vi "Init Device.vi"(7 "Layout Ref":refnum<vi>, 8 "error in (no error)":errorcluster, 10 "Chan# Array":i32[](array[numeric])=[4, 16] caption="#AOs [0,8]   #DOs [0,32]", 11 "NI Card in":refnum<class "NI Card.lvclass">) -> (0 "error out":errorcluster={"status"=TRUE, "code"=1055, "source"="Property Node in NI Card.lvclass:Init Device.vi"}, 3 "NI Card out":refnum<class "NI Card.lvclass">)   [LabVIEW 2013, in "NI Card.lvclass"]
doc: "Initialize the correct columns and their default appearance.\nUse the front panel to change default appearance of the device in the Add/Manage devices.\n\nThe (optional) Chan# Array, used for Old version loading, is [# AOs, # DOs]."
uses:
  NI Card.lvclass
  TypeDefs/DigitalColumnAppearCluster.ctl
  TypeDefs/ColumnAppearCluster.ctl
  ColumnVIs/Column/Column.lvclass
  ColumnVIs/DigitalCol/DigitalCol.lvclass
  NI Card.lvclass/NI Card.ctl
panel:
  in  "AI Default Name":string
  in  "Analog Column Defaults":T1={"Column Name"="", "Width"=30, "Bkgd"=[16448250], "Text"=[0]}
  in  "Num AIs":i32
  in  "Digital Column Defaults":T2={"Column Name"="", "Width"=15, "Bkgd"=[1985280, 6618880, 14090026], "Text"=[16448250, 0, 0]}
  # "Num AOs, DOs are coerced on Block diagram to be in shown range.\nMUST include at least 1 to configure each column type."
  # "The choices you make here dictate what will appear when you Add an 'NI card' device.\nPick default widths, colors, (column names) and numbers of channels.\nThen go to the menu Edit >> Make Current Values Default and re-save the VI."
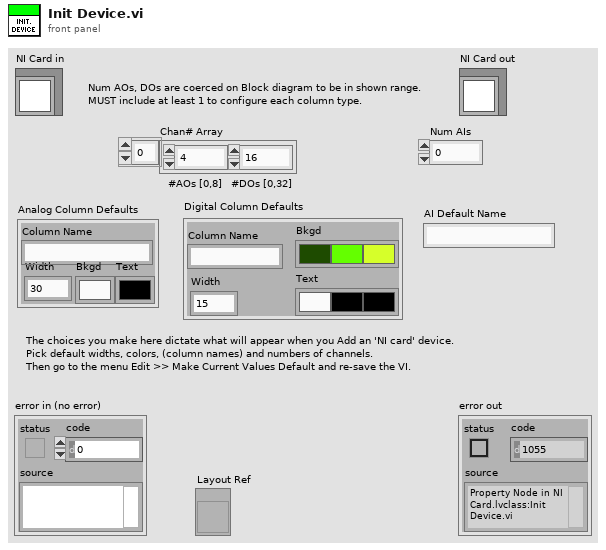
[diagram p1: front panel]
types:
  T1 = typedef "ColumnAppearCluster.ctl" = cluster{"Column Name":string, "Width":u32, "Bkgd":u32[], "Text":u32[]}
  T2 = typedef "DigitalColumnAppearCluster.ctl" = cluster{"Column Name":string, "Width":u32, "Bkgd":u32[], "Text":u32[]}
  T3 = cluster{"DAQmx Global Channel":refnum<k21>, "AI Default Name":string}
  T4 = cluster{"DAQmx Global Channel":refnum<k21>, "Column Name":string}
  T5 = cluster{"DAQmx Global Channel":refnum<k21>, "Column Name":string}[]
  T6 = cluster{"DAQmx Global Channel":refnum<k21>, "AI Default Name":string}[]
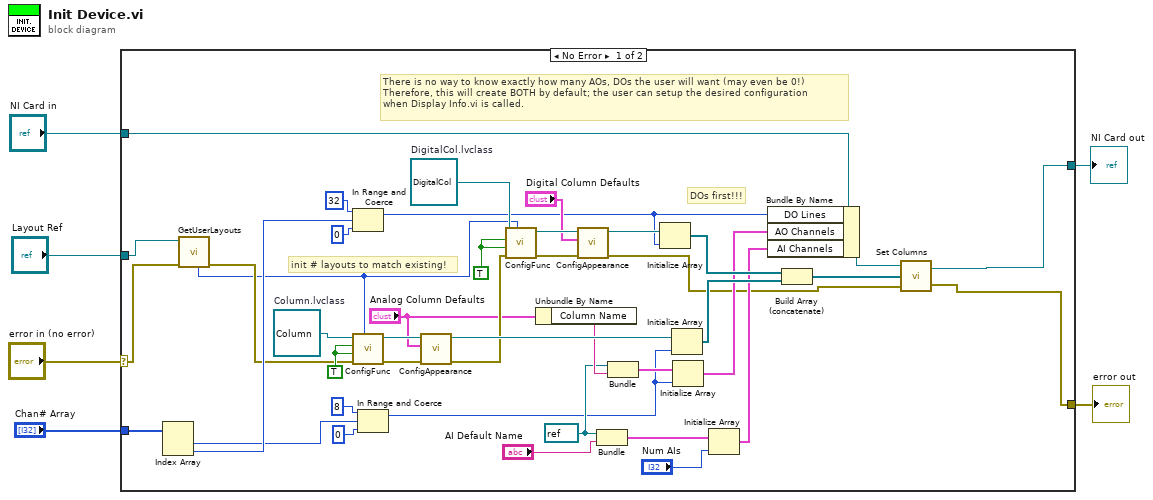
[diagram p0: block diagram]
diagram:
  n1 = case shown="No Error" "error in (no error)" {
    selector: "error in (no error)" -> [w12 w49]
    tunnel: "NI Card in" -> [w48 w50]
    tunnel: [w8 w50] -> w4
    tunnel: [w7 w49] -> w3
    tunnel: "Layout Ref" -> [w9 _]
    tunnel: "Chan# Array" -> [w15 _]
    frame No Error {
      w28 = refnum<k21> refnum ("DAQmx Global Channel")
      w45 = TRUE ("Disableable? (True)")
      w46 = TRUE ("Disableable? (True)")
      w47 = refnum<class "DigitalCol.lvclass"> refnum  # DigitalCol.lvclass
      w44 = refnum<class "Column.lvclass"> refnum  # Column.lvclass
      # "init # layouts to match existing!"
      # "DOs first!!!"
      # "There is no way to know exactly how many AOs, DOs the user will want (may even be 0!)\nTherefore, this will create BOTH by default; the user can setup the desired configuration\nwhen Display Info.vi is called."
      n2 = Index Array(array=w15) -> (element #1=w13:i32, element #2=w14:i32)  [unwired: 2 in]
      n3 = call "GetUserLayouts.vi"("error in (no error)"=w12, "Layout Ring Refnum"=w9) -> ("error out"=w11:errorcluster, "Num User Layouts"=w10:i32)  [unwired: 5 in, 3 out]
      n4 = In Range and Coerce(upper limit=32, x=w14, lower limit=0) -> (coerced(x)=w21:i32)  [unwired: 1 out]
      n5 = call "ConfigFunc.vi"("Num Layouts (ignored)"=w10, "error in (no error)"=w11, "isVariable? (True)"=w45, "Disableable? (True)"=w45, "Column in"=w44) -> ("error out"=w35:errorcluster, "Column out"=w37:refnum<class "Column.lvclass">)  [unwired: 5 in]
      n6 = In Range and Coerce(upper limit=8, x=w13, lower limit=0) -> (coerced(x)=w16:i32)  [unwired: 1 out]
      n7 = call "ConfigAppearance.vi"("error in (no error)"=w35, "Column Appearance"="Analog Column Defaults", "Column in"=w37) -> ("error out"=w34:errorcluster, "Column out"=w36:refnum<class "Column.lvclass">)  [unwired: 7 in]
      n8 = call "ConfigFunc.vi"("Num Layouts (ignored)"=w10, "error in (no error)"=w34, "isVariable? (True)"=w46, "Disableable? (True)"=w46, "Column in"=w47) -> ("error out"=w39:errorcluster, "Column out"=w41:refnum<class "DigitalCol.lvclass">)  [unwired: 5 in]
      n9 = Unbundle By Name("Analog Column Defaults") -> ("Column Name"=w29:string)
      n10 = call "ConfigAppearance.vi"("error in (no error)"=w39, "Column Appearance"="Digital Column Defaults", "Column in"=w41) -> ("error out"=w22:errorcluster, "Column out"=w40:refnum<class "DigitalCol.lvclass">)  [unwired: 7 in]
      n11 = Bundle("DAQmx Global Channel"=w28, "AI Default Name"="AI Default Name") -> (w30:T3)  [unwired: 1 in]
      n12 = Bundle("DAQmx Global Channel"=w28, "Column Name"=w29) -> (w27:T4)  [unwired: 1 in]
      n13 = Initialize Array(w40, w21) -> (w43:refnum<class "DigitalCol.lvclass">[])
      n14 = Initialize Array(w36, w16) -> (w42:refnum<class "Column.lvclass">[])
      n15 = Initialize Array(w27, w16) -> (w26:T5)
      n16 = Initialize Array(w30, "Num AIs") -> (w25:T6)
      n17 = Bundle By Name(cluster=w48, "DO Lines"=w21, "AO Channels"=w26, "AI Channels"=w25) -> (w24:refnum<class "NI Card.lvclass">)
      n18 = Build Array (concatenate)(w43, w42) -> (w23:refnum<class "Column.lvclass">[])
      n19 = call-dynamic "Set Columns.vi"("error in (no error)"=w22, "Columns"=w23, "NI Card in"=w24) -> ("error out"=w7:errorcluster, "NI Card out"=w8:refnum<class "NI Card.lvclass">)  [unwired: 1 in]
    }
    frame Error {
    }
  }
  "error out" <- w3
  "NI Card out" <- w4
